vi "Labo2.1.vi"() -> ()   [LabVIEW 2020]
panel:
  in  "stop 2":bool
  out "wynik 4":string
  out "wynik 3":string
  out "wynik 2":string
  out "wynik 1":string
  out "wartosc 4":dbl
  out "wartosc 3":dbl
  out "wartosc 2":dbl
  out "wartosc 1":dbl
  out "bs4":string
  out "bs3":string
  out "bs 2":string
  out "bs1":string
  in  "B 8":dbl
  in  "B4":dbl
  in  "B3":dbl
  in  "B7":dbl
  in  "B6":dbl
  in  "B2":dbl
  in  "B 1":dbl
  in  "B5":dbl
  out "oper 4":string
  out "oper 3":string
  out "oper 2":string
  out "oper 1":string
  out "as4":string
  out "as3":string
  out "as2":string
  out "as1":string
  in  "A 8":dbl
  in  "A 4":dbl
  in  "A 3":dbl
  in  "A7":dbl
  in  "A6":dbl
  in  "A 2":dbl
  in  "A 1":dbl
  in  "A 5":dbl
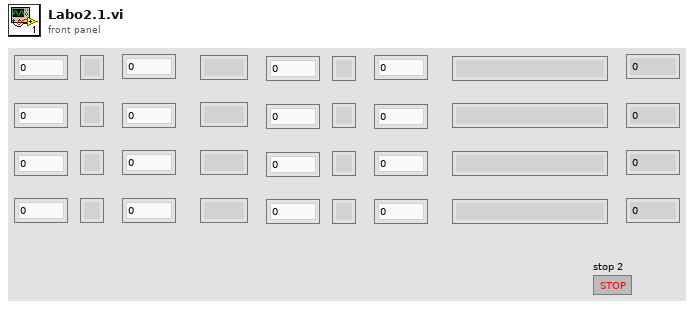
[diagram p1: front panel]
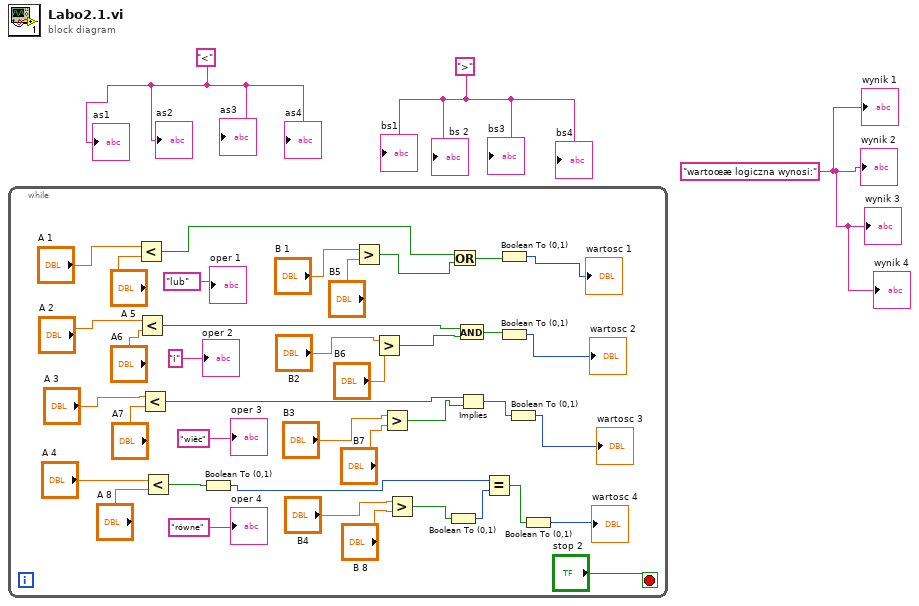
[diagram p0: block diagram]
diagram:
  w3 = "wartoœæ logiczna wynosi:"
  w1 = "<"
  w2 = ">"
  n1 = while {
    stop <- "stop 2" stop-if-true
    n2 = Less?(x="A 1", y="A 5") -> (x < y?=w20:bool)
    n3 = Less?(x="A 2", y="A6") -> (x < y?=w18:bool)
    n4 = Less?(x="A 3", y="A7") -> (x < y?=w22:bool)
    n5 = Less?(x="A 4", y="A 8") -> (x < y?=w10:bool)
    n6 = Boolean To (0,1)(Boolean=w10) -> (0, 1=w8:i16)
    n7 = Greater?(x="B 1", y="B5") -> (0:w19:bool)
    n8 = Greater?(x="B2", y="B6") -> (0:w17:bool)
    n9 = Greater?(x="B3", y="B7") -> (0:w21:bool)
    n10 = Greater?(x="B4", y="B 8") -> (0:w9:bool)
    n11 = Boolean To (0,1)(Boolean=w9) -> (0, 1=w7:i16)
    n12 = Or(x=w20, y=w19) -> (x .or. y?=w16:bool)
    n13 = And(x=w18, y=w17) -> (x .and. y?=w14:bool)
    n14 = Implies(1:w21, 2:w22) -> (0:w12:bool)
    n15 = Equal?(x=w8, y=w7) -> (x = y?=w6:bool)
    n16 = Boolean To (0,1)(Boolean=w16) -> (0, 1=→"wartosc 1":i16)
    n17 = Boolean To (0,1)(Boolean=w14) -> (0, 1=→"wartosc 2":i16)
    n18 = Boolean To (0,1)(Boolean=w12) -> (0, 1=→"wartosc 3":i16)
    n19 = Boolean To (0,1)(Boolean=w6) -> (0, 1=→"wartosc 4":i16)
    "oper 1" <- "lub"
    "oper 2" <- "i"
    "oper 3" <- "wiêc"
    "oper 4" <- "równe"
  }
  "as1" <- w1
  "as2" <- w1
  "as3" <- w1
  "as4" <- w1
  "bs1" <- w2
  "bs 2" <- w2
  "bs3" <- w2
  "bs4" <- w2
  "wynik 1" <- w3
  "wynik 2" <- w3
  "wynik 3" <- w3
  "wynik 4" <- w3
